vi "Copy Audio Sample.vi"(8 "error in (no error)":errorcluster, 9 "Length":i32, 10 "Offset":i32, 11 "Deck in":refnum<class "Sample.lvclass">) -> (0 "error out":errorcluster, 2 "Audio Block":dbl[][](array[numeric]), 3 "Deck out":refnum<class "Sample.lvclass">)   [LabVIEW 2020, in "Sample.lvclass"]
doc: "Copy a sample block of audio from the DVR based on Offset and Length. If Offset + Length exceeds the size of audio in the DVR, the sample buffer is zero padded.\n\nLength can be negative or positive. If length is negative, the sample data returned is reversed."
uses:
  Sample.lvclass
  Sample.lvclass/Sample.ctl
  Packed Libraries/Audio Processing.lvlibp
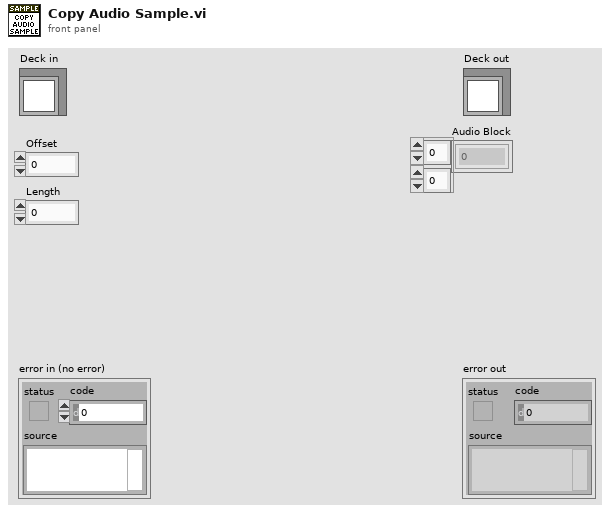
[diagram p1: front panel]
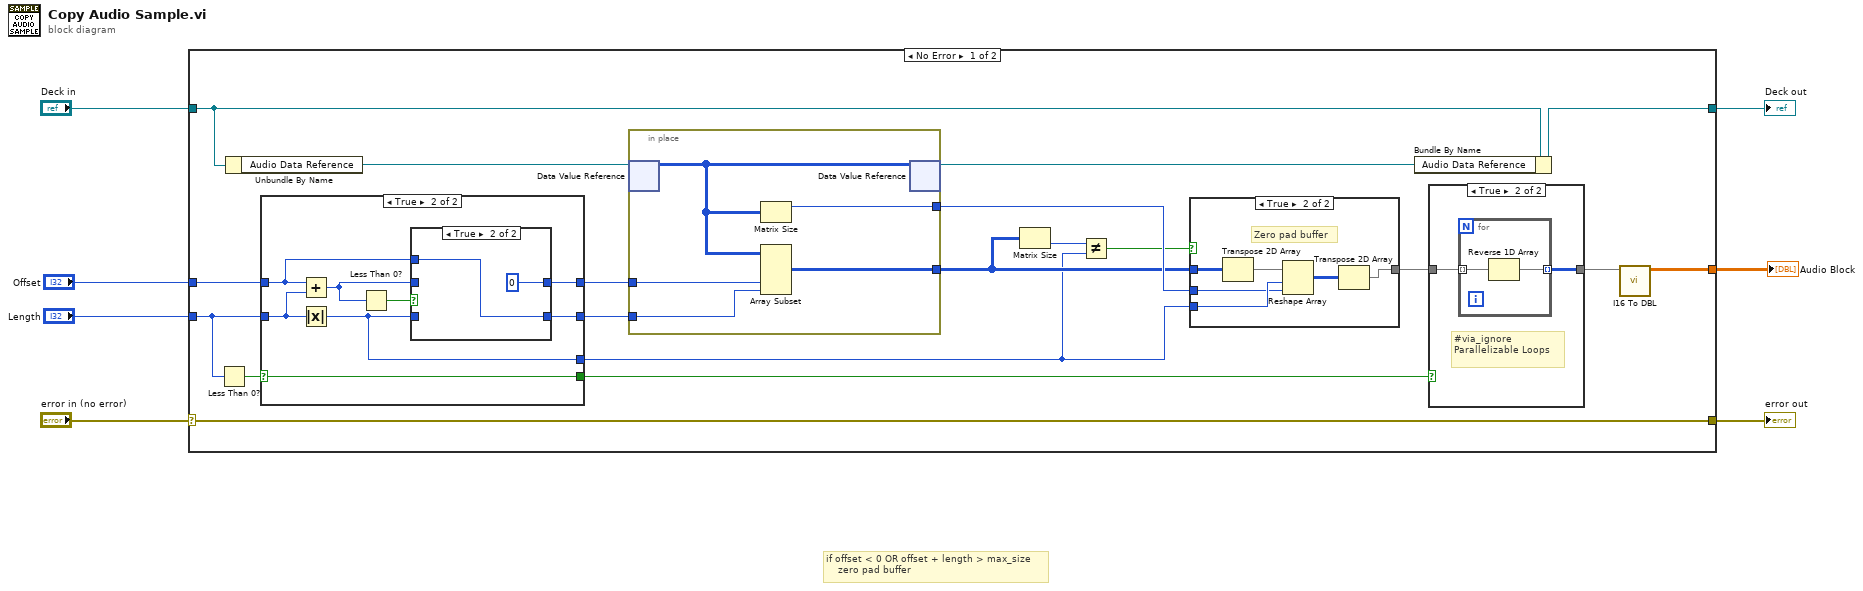
[diagram p0: block diagram]
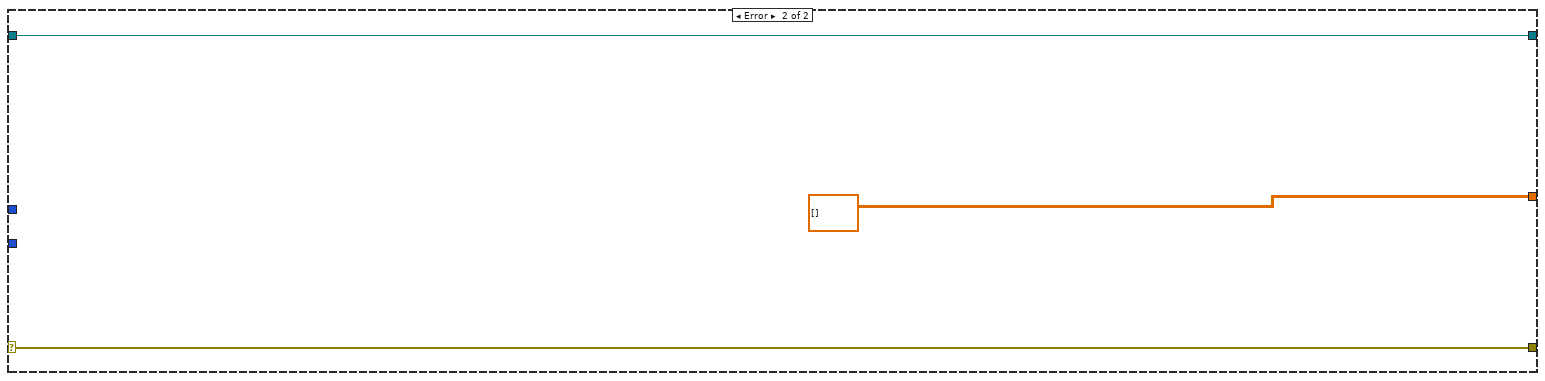
[diagram p6: hidden frame]
diagram:
  # "if offset < 0 OR offset + length > max_size\n    zero pad buffer"
  n1 = case shown="No Error" "error in (no error)" {
    selector: "error in (no error)" -> [w26 w61]
    tunnel: [w26 w61] -> w5
    tunnel: [w23 w60] -> w4
    tunnel: "Deck in" -> [w22 w60]
    tunnel: "Offset" -> [w20 _]
    tunnel: "Length" -> [w18 _]
    tunnel: [w16 dbl[][] []] -> w1
    frame No Error {
      n2 = Less Than 0?(x=w18) -> (x < 0?=w21:bool)
      n3 = Unbundle By Name(w22) -> ("Audio Data Reference"=w25:refnum<data-value>)
      n4 = case shown="True" w21 {
        selector: w21 -> [w40 w48]
        tunnel: [w41 w45] -> w12
        tunnel: w20 -> [w41 w43]
        tunnel: [w39 w44] -> w19
        tunnel: w18 -> [w39 w49]
        tunnel: [w40 w48] -> w13
        tunnel: [w39 w42] -> w9
        frame False {
        }
        frame True {
          n5 = Add(x=w43, y=w49) -> (x+y=w46:i32)
          n6 = Absolute Value(x=w49) -> (abs(x)=w42:i32)
          n7 = Less Than 0?(x=w46) -> (x < 0?=w47:bool)
          n8 = case shown="True" w47 {
            tunnel: w46 -> [w51 _]
            tunnel: [w51 0] -> w45
            tunnel: w42 -> [w50 _]
            tunnel: [w50 w53] -> w44
            tunnel: w43 -> [_ w53]
            frame False {
            }
            frame True {
            }
          }
        }
      }
      n9 = in-place {
        in-place-border: w19 -> [w58]
        in-place-border: w12 -> [w57]
        in-place-border: [w55] -> w14
        in-place-border: [w54] -> w11
        n10 = in-place-dvr #1(w25) -> (w56:i16[][])  [unwired: 1 out]
        n11 = Matrix Size(0:w56) -> (1:w55:i32)  [unwired: 1 out]
        n12 = Array Subset(array=w56, index (col)=w57, length (col)=w58) -> (w54:i16[][])  [unwired: 2 in]
        n13 = in-place-dvr #1(w56) -> (w24:refnum<data-value>)  [unwired: 1 out]
      }
      n14 = Matrix Size(0:w11) -> (2:w10:i32)  [unwired: 1 out]
      n15 = Not Equal?(x=w10, y=w9) -> (x != y?=w8:bool)
      n16 = case shown="True" w8 {
        tunnel: w11 -> [w27 w31]
        tunnel: w14 -> [_ w28]
        tunnel: w9 -> [_ w29]
        tunnel: [w27 w30] -> w15
        frame False {
        }
        frame True {
          # "Zero pad buffer"
          n17 = Transpose 2D Array(2D array=w31) -> (transposed array=w33:i16[][])
          n18 = Reshape Array(w33, w29, w28) -> (w32:i16[][])
          n19 = Transpose 2D Array(2D array=w32) -> (transposed array=w30:i16[][])
        }
      }
      n20 = Bundle By Name(cluster=w22, "Audio Data Reference"=w24) -> (w23:refnum<class "Sample.lvclass">)
      n21 = case shown="True" w13 {
        tunnel: [w34 w35] -> w17
        tunnel: w15 -> [w34 w36]
        frame False {
        }
        frame True {
          # "#via_ignore Parallelizable Loops"
          n22 = for {
            tunnel: w36 -> [w38] mode=indexing
            tunnel: [w37] -> w35 mode=indexing
            n23 = Reverse 1D Array(array=w38) -> (reversed array=w37:i16[])
          }
        }
      }
      n24 = call "I16 To DBL.vi"("Audio Data (2D I16)"=w17) -> ("Audio Data (2D DBL)"=w16:dbl[][])  [unwired: 9 in, 1 out]
    }
    frame Error {
    }
  }
  "error out" <- w5
  "Deck out" <- w4
  "Audio Block" <- w1
